vi "JKISM++ Config Array Parameter Cache Size.vi"(2 "size(1M)":i32=1000000 format="%.0p") -> ()   [LabVIEW 2020, in "JKISM++ Array Parameter Support.lvlib"]
doc: "Convert complex argument(variant) to hex string, which could be safely used as state argument without broking the string queue logic.\n\n<b>Inputs:</b>\n - <b>Variant</b>: Complex data in variant format.\n\n<b>Outputs:</b>\n - <b>HEX String (0-9,A-F)</b>: Hex String, which contains no invisible string following JKISM's rule"
uses:
  _support/Operation-FGV-MassData.ctl
  JKISM++ Array Parameter Support.lvlib
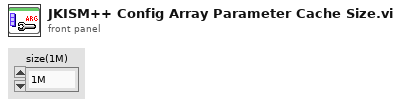
[diagram p1: front panel]
types:
  T1 = typedef "JKISM++ Array Parameter Support.lvlib/Operation-FGV-MassData.ctl" = enum16{"Initialize", "Read", "Write", "Status", "Release"}
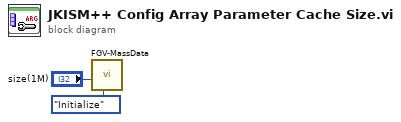
[diagram p0: block diagram]
diagram:
  n1 = call "FGV-MassData.vi"("Operation"=Operation-FGV-MassData."Initialize", "size"="size(1M)") -> ()  [unwired: 6 in, 4 out]
